vi "Add Object Parameter - 1D Array Double.vi"(8 "error in (no error)":errorcluster, 9 "Name":string, 10 "1D Double":dbl[](array[numeric]), 11 "JSON Tree in (JSON Object)":variant) -> (0 "error out":errorcluster, 3 "JSON Tree out (JSON Object)":variant)   [LabVIEW 2013, in "i3-json.lvlib"]
doc: "Adds a 1D Numeric array to the JSON Tree"
uses:
  i3-json.lvlib
  JSON Types/JSON Type.ctl
  JSON Types/JSON Compatible Type.ctl
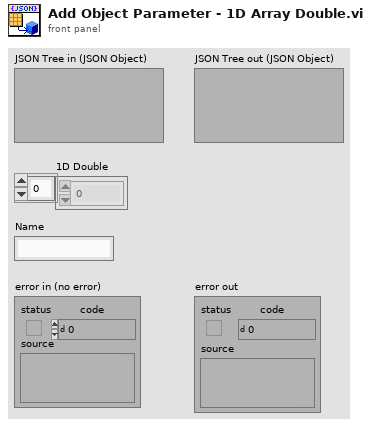
[diagram p1: front panel]
types:
  T1 = typedef "i3-json.lvlib/JSON Compatible Type.ctl" = enum16{"1D Double Array", "1D String Array", "1D Boolean Array", "Unknown"}
  T2 = typedef "i3-json.lvlib/JSON Type.ctl" = enum8{"JSON Compatible", "JSON Array", "JSON Object", "JSON Null", "Double", "String", "Boolean", "Unknown"}
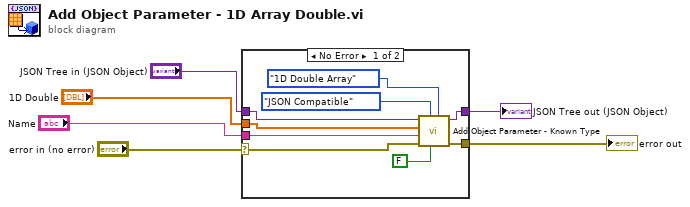
[diagram p0: block diagram]
diagram:
  n1 = case shown="No Error" "error in (no error)" {
    selector: "error in (no error)" -> [w9 w17]
    tunnel: [w15 w17] -> w5
    tunnel: [w14 w16] -> w4
    tunnel: "JSON Tree in (JSON Object)" -> [w13 w16]
    tunnel: "1D Double" -> [w8 _]
    tunnel: "Name" -> [w7 _]
    frame No Error {
      n2 = call "Add Object Parameter - Known Type.vi"("JSON Compatible Type"=JSON_Compatible_Type."1D Double Array", "Add Parameter as JSON Tree?"=FALSE, "JSON Type"=JSON_Type."JSON Compatible", "error in (no error)"=w9, "Name"=w7, "Value"=w8, "JSON Tree in (JSON Object)"=w13) -> ("error out"=w15:errorcluster, "JSON Tree out (JSON Object)"=w14:variant)  [unwired: 3 in]
    }
    frame Error {
    }
  }
  "error out" <- w5
  "JSON Tree out (JSON Object)" <- w4
